vi "6_1_sub_arecharequal.vi"(11 "Array in":string[](array[string])) -> (0 "indices of removed elements":i32[](array[numeric]))   [LabVIEW 2025, in "2022.lvlib"]
uses:
  2022.lvlib
  <userlib>/_OpenG.lib/array/array.llb/Remove Duplicates from 1D Array (String)__ogtk.vi
  <userlib>/_OpenG.lib/array/array.llb/openg_array.lvlib
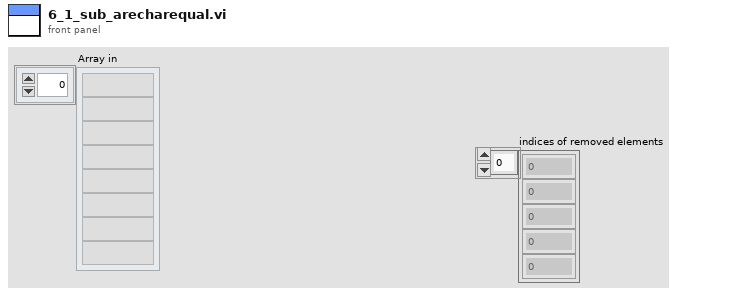
[diagram p1: front panel]
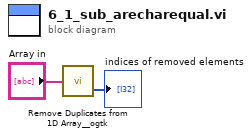
[diagram p0: block diagram]
diagram:
  n1 = call-poly <userlib>:"Remove Duplicates from 1D Array__ogtk.vi"("Input Array"="Array in") -> ("indices of removed elements"=→"indices of removed elements":i32[])  [unwired: 1 out]
